vi "check_keithley-2450_is_connected.vi"() -> (0 "error out":errorcluster)   [LabVIEW 2016]
panel:
  out "standard output":string
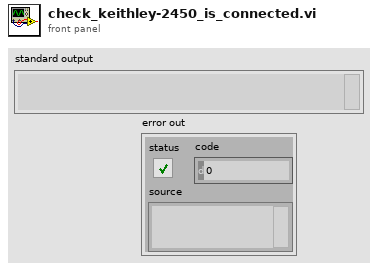
[diagram p1: front panel]
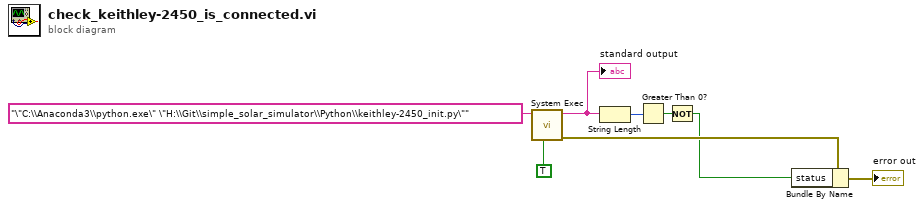
[diagram p0: block diagram]
diagram:
  n1 = call <vilib>:"System Exec.vi"("run minimized? (F)"=TRUE, "command line"="\"C:\\Anaconda3\\python.exe\" \"H:\\Git\\simple_solar_simulator\\Python\\keithley-2450_init.py\"") -> ("error out"=w3:errorcluster, "standard output"=w6:string)  [unwired: 6 in, 2 out]
  "standard output" <- w6
  n2 = String Length(string=w6) -> (length=w5:i32)
  n3 = Greater Than 0?(x=w5) -> (x > 0?=w4:bool)
  n4 = Not(x=w4) -> (.not. x?=w1:bool)
  n5 = Bundle By Name(cluster=w3, "status"=w1) -> (→"error out":errorcluster)
